vi "Repack Pixels_Pixel Bus to FIFO U16x8.vi"(10 "Input Valid":bool=TRUE, 11 "Pixel Bus In":T1={"Pixel Data"=[0, 0, 0, 0, 0, 0, 0, 0], "DV"=[FALSE, FALSE, FALSE, FALSE, FALSE, FALSE, FALSE, FALSE], "EOL"=FALSE, "EOI"=FALSE, "Data Type"=enum."U16 x 8"}) -> (2 "Output Valid":bool, 3 "output array":u16[](array[numeric]))   [LabVIEW 2017, in "NI_VDM_FPGA_Basics.lvlib"]
uses:
  <vilib>/visionFPGA/NI_VDM_FPGA_Basics.lvlib
  <vilib>/visionFPGA/Controls/IMAQ FPGA Pixel Bus u16x8.ctl
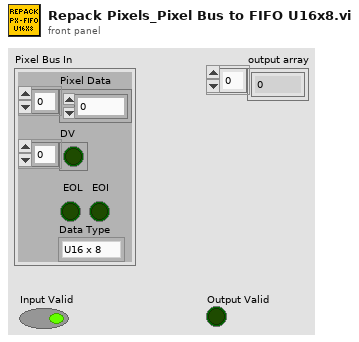
[diagram p1: front panel]
types:
  T1 = typedef "IMAQ FPGA Pixel Bus u16x8.ctl" = cluster{"Pixel Data":u16[], "DV":bool[], "EOL":bool, "EOI":bool, "Data Type":enum16{"U16 x 8"}}
  T2 = cluster{"Pixel Data":u16[], "DV":bool[], "EOL":bool, "EOI":bool, "Data Type":enum16{"U16 x 8"}}
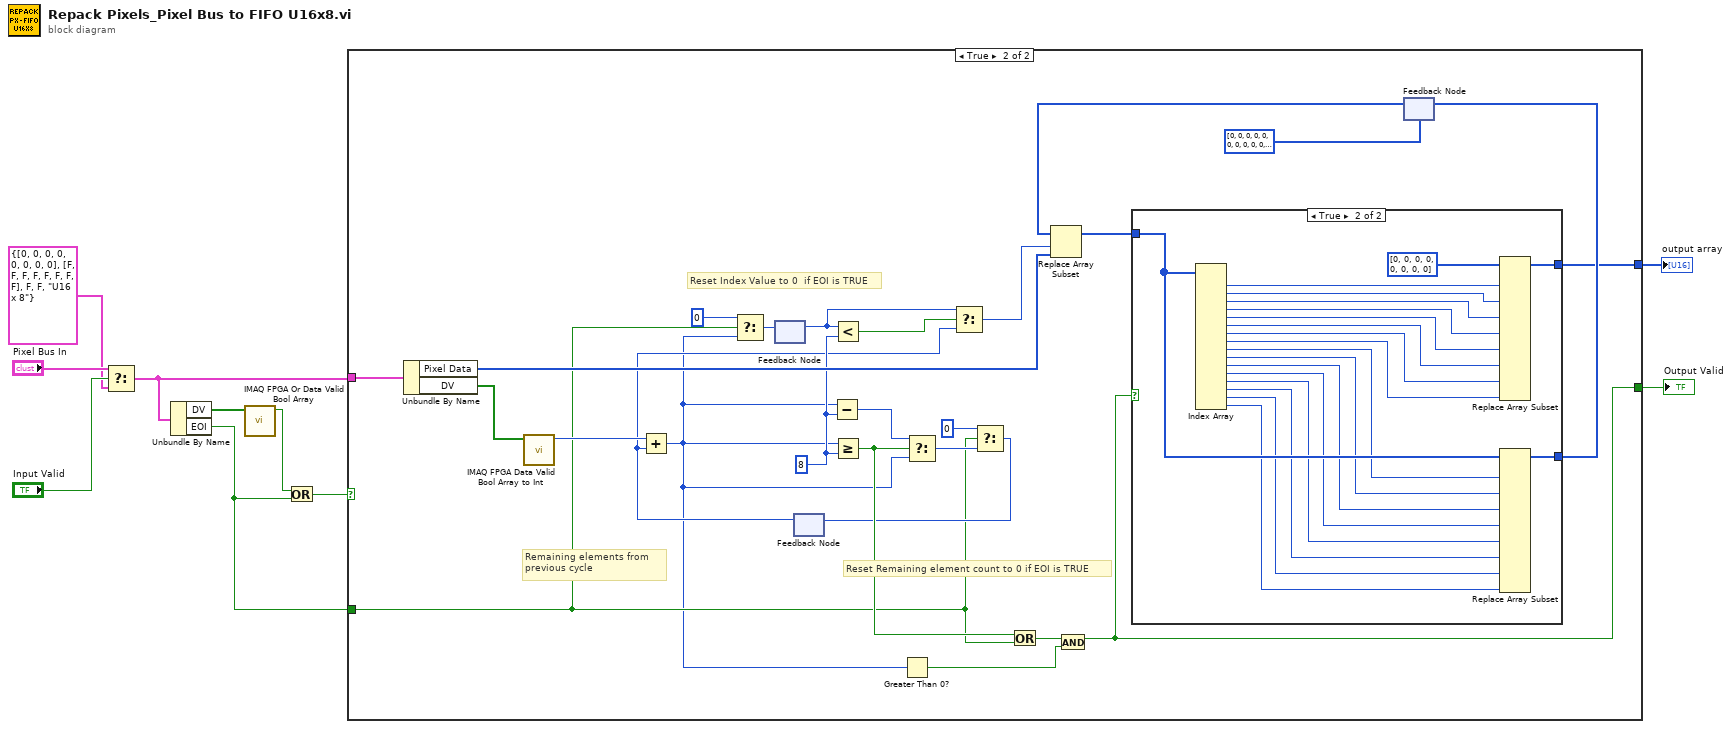
[diagram p0: block diagram]
diagram:
  n1 = Select(t="Pixel Bus In", s="Input Valid", f=T2 {"Pixel Data"=[0, 0, 0, 0, 0, 0, 0, 0], "DV"=[FALSE, FALSE, FALSE, FALSE, FALSE, FALSE, FALSE, FALSE], "EOL"=FALSE, "EOI"=FALSE, "Data Type"=enum."U16 x 8"}) -> (s? t:f=w5:T1)
  n2 = Unbundle By Name(w5) -> ("DV"=w4:bool[], "EOI"=w1:bool)
  n3 = call <vilib>:"IMAQ FPGA Or Data Valid Bool Array.vi"("DV Array In"=w4) -> ("DV Out"=w3:bool)  [unwired: 10 in]
  n4 = Or(x=w3, y=w1) -> (x .or. y?=w8:bool)
  n5 = case shown="True" w8 {
    tunnel: w5 -> [_ w36]
    tunnel: [_ w30] -> w10
    tunnel: [_ w13] -> w9
    tunnel: w1 -> [_ w14]
    frame False {
    }
    frame True {
      w28 = u16 8 ("y")
      # "Reset Remaining element count to 0 if EOI is TRUE"
      # "Reset Index Value to 0  if EOI is TRUE"
      # "Remaining elements from \nprevious cycle"
      n6 = Unbundle By Name(w36) -> ("Pixel Data"=w32:u16[], "DV"=w23:bool[])
      n7 = call <vilib>:"IMAQ FPGA Data Valid Bool Array to Int.vi"("DV In"=w23) -> ("Sum DV Out"=w22:u8)  [unwired: 10 in]
      n8 = feedback #1() -> (w27:u16)  [unwired: 1 in]
      n9 = feedback #2() -> (w21:u16)  [unwired: 1 in]
      n10 = Add(x=w22, y=w21) -> (x+y=w12:u16)
      n11 = Select(t=u16 0, s=w14, f=w12) -> (s? t:f=w16:u16)
      n12 = feedback-in #1(w16) -> ()
      n13 = Subtract(x=w12, y=w28) -> (x-y=w29:u16)
      n14 = Less?(x=w27, y=w28) -> (x < y?=w25:bool)
      n15 = Greater Or Equal?(x=w12, y=w28) -> (x >= y?=w24:bool)
      n16 = Greater Than 0?(x=w12) -> (x > 0?=w11:bool)
      n17 = Select(t=w29, s=w24, f=w12) -> (s? t:f=w19:u16)
      n18 = Select(t=w27, s=w25, f=w21) -> (s? t:f=w26:u16)
      n19 = Select(t=u16 0, s=w14, f=w19) -> (s? t:f=w17:u16)
      n20 = feedback-in #2(w17) -> ()
      n21 = Or(x=w24, y=w14) -> (x .or. y?=w20:bool)
      n22 = And(x=w20, y=w11) -> (x .and. y?=w13:bool)
      n23 = feedback #3(u16[] [0, 0, 0, 0, 0, 0, 0, 0, 0, 0, 0, 0, 0, 0, 0, 0] ("Pixel Data")) -> (w33:u16[])
      n24 = Replace Array Subset(array=w33, new element=w32, index=w26) -> (w31:u16[])
      n25 = case shown="True" w13 {
        tunnel: [w37 w57] -> w34
        tunnel: w31 -> [w37 w56]
        tunnel: [_ w38] -> w30
        frame False {
        }
        frame True {
          n26 = Index Array(array=w56) -> (element #1=w54:u16, element #2=w53:u16, element #3=w52:u16, element #4=w51:u16, element #5=w50:u16, element #6=w49:u16, element #7=w48:u16, element #8=w47:u16, element #9=w46:u16, element #10=w45:u16, element #11=w44:u16, element #12=w43:u16, element #13=w42:u16, element #14=w41:u16, element #15=w40:u16, element #16=w39:u16)  [unwired: 16 in]
          n27 = Replace Array Subset(array=u16[] [0, 0, 0, 0, 0, 0, 0, 0] ("Pixel Data"), new element #1=w54, new element #2=w53, new element #3=w52, new element #4=w51, new element #5=w50, new element #6=w49, new element #7=w48, new element #8=w47) -> (w38:u16[])  [unwired: 8 in]
          n28 = Replace Array Subset(array=w56, new element #1=w46, new element #2=w45, new element #3=w44, new element #4=w43, new element #5=w42, new element #6=w41, new element #7=w40, new element #8=w39) -> (w57:u16[])  [unwired: 8 in]
        }
      }
      n29 = feedback-in #3(w34) -> ()
    }
  }
  "output array" <- w10
  "Output Valid" <- w9
